vi "Pfeiffer Vacuum ModulLine Read Data.vi"(8 "error in (no error)":errorcluster, 9 "PV ModulLine-Cluster":T1={"Parameter"=enum." Pressure  [mbar] (740)", "Parameter\nread only<->describe"=FALSE, "Correction facktor\n(0,20 - 9,90) "=1.0} {"Correction facktor\n(0,20 - 9,90)" min=0.2 max=9.9 step=0.01 format="%.2f"}, 10 "Adress of unit":u16=10 min=1 max=999 step=1, 11 "VISA session in":refnum<visa-resource-name>) -> (0 "error out":errorcluster, 3 "response (data)":string)   [LabVIEW 2021]
doc: "This VI is an example of how to use the Pfeiffer Vacuum subVIs programmatically. This VI first initializes the instrument, takes measurements, then closes the instrument."
uses:
  <instrlib>/Pfeiffer Vacuum/Public/ModulLine/PV ModulLine - Cluster.ctl
  <instrlib>/Pfeiffer Vacuum/Pfeiffer Vacuum.lvlib
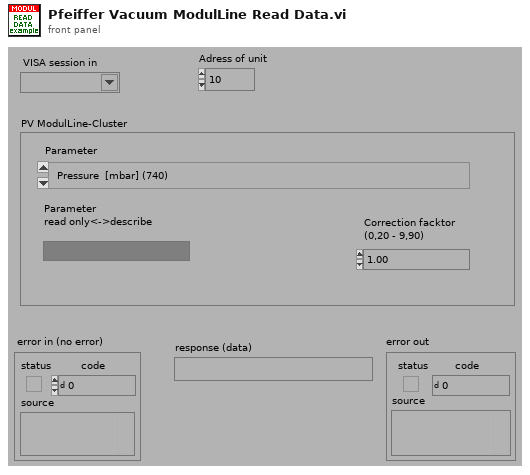
[diagram p1: front panel]
types:
  T1 = typedef "Pfeiffer Vacuum.lvlib/PV ModulLine - Cluster.ctl" = cluster{"Parameter":enum16{" Pressure  [mbar] (740)", " Correction factor sensor (742)", " Actual error code (read only) (303)", " Software version Transmitter (read only) (312)", " Unit type Transmitter (read only) (349)"}, "Parameter\nread only<->describe":bool, "Correction facktor\n(0,20 - 9,90) ":sgl}
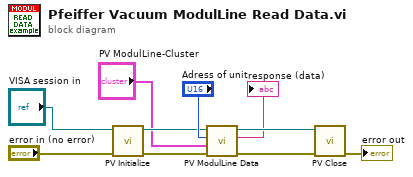
[diagram p0: block diagram]
diagram:
  n1 = call <instrlib>:"PV Initialize.vi"("error in (no error)"="error in (no error)", "VISA session in"="VISA session in") -> ("error out"=w4:errorcluster, "VISA session out"=w3:refnum<visa-resource-name>)  [unwired: 8 in]
  n2 = call <instrlib>:"PV ModulLine Data.vi"("error in (no error)"=w4, "PV ModulLine-Cluster"="PV ModulLine-Cluster", "Adress of unit"="Adress of unit", "VISA session"=w3) -> ("error out"=w10:errorcluster, "response (data)"=→"response (data)":string, "dup VISA session"=w9:refnum<visa-resource-name>)  [unwired: 5 in]
  n3 = call <instrlib>:"PV Close.vi"("VISA session"=w9, "error in (no error)"=w10) -> ("error out"=→"error out":errorcluster)  [unwired: 13 in]
